vi "NI VeriStand - Set Fault Value.vi"(8 "error in (no error)":errorcluster, 9 "Fault Value":dbl, 10 "Channel":string, 11 "ChannelFault in":T1) -> (0 "error out":errorcluster, 3 "ChannelFault out":T1)   [LabVIEW 2020, in "NI_VS ChannelFault ExecutionAPI.lvlib"]
doc: "Sets the fault value of the specified channel."
uses:
  <vilib>/NI VeriStand/Execution/ChannelFaultManager/NI_VS ChannelFault ExecutionAPI.lvlib
  <vilib>/NI VeriStand/Execution/ChannelFaultManager/ChannelFaultAPI.ctl
  NationalInstruments.VeriStand.ClientAPI
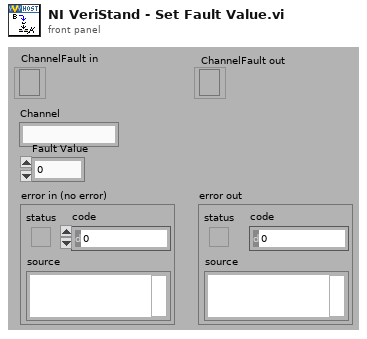
[diagram p1: front panel]
types:
  T1 = typedef "NI_VS ChannelFault ExecutionAPI.lvlib/ChannelFaultAPI.ctl" = refnum<k24>
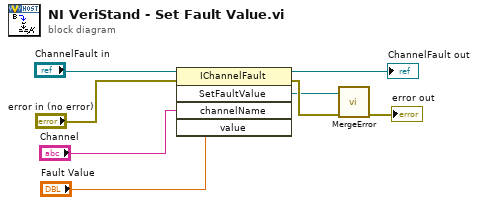
[diagram p0: block diagram]
diagram:
  n1 = invoke class="IChannelFault" method="SetFaultValue"(reference="ChannelFault in", error in="error in (no error)", "channelName"="Channel", "value"="Fault Value") -> (reference out=→"ChannelFault out":T1, error out=w6:errorcluster, "SetFaultValue"=w5:refnum<k24>)  [unwired: 1 in, 2 out]
  n2 = call <vilib>:"MergeError.vi"("error in (no error)"=w6, "Error"=w5) -> ("error out"=→"error out":errorcluster)  [unwired: 9 out]
